vi "Grab Tool.vi"(8 "error in":errorcluster, 9 "Tool Type":enum16{"Stamp", "Weight"}(ring), 10 "Slot Number":i32, 11 "GrabberTool in":refnum<class "GrabberTool Class.lvclass">) -> (0 "error out":errorcluster, 3 "GrabberTool out":refnum<class "GrabberTool Class.lvclass">)   [LabVIEW 2011, in "GrabberTool Class.lvclass"]
uses:
  GrabberTool Class.lvclass
  Config Manager Class/Type Definitions/Part Type.ctl
  Config Manager Class/Type Definitions/Offset.ctl
  Config Manager Class/Type Definitions/Named Position.ctl
  WorkTable Class/WorkTable Class.lvclass
  Vec3d Class/Vec3d Class.lvclass
  Config Manager Class/Read Geometry Definition 3D.vi
  Config Manager Class/Config Manager Class.lvclass
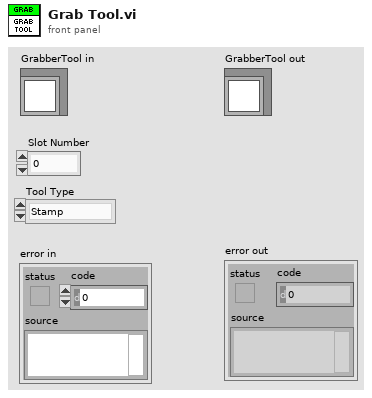
[diagram p1: front panel]
types:
  T1 = typedef "Part Type.ctl" = enum16{"BBM", "HDI", "BARE HDI", "GLUERESERVOIR", "STAMP_1", "STAMP_2", "STAMP_3", "STAMP_4", "STAMP_5", "WEIGHT_1", "WEIGHT_2", "WEIGHT_3", "WEIGHT_4", "WEIGHT_5", "WEIGHT_6", "WEIGHT_7", "WEIGHT_8", "PICKER_TOOL", "GRABER_TOOL"}
  T2 = typedef "Offset.ctl" = enum16{"needle_offset", "tool_holder_offset"}
  T3 = typedef "Named Position.ctl" = enum16{"home", "module_chuck_0", "module_chuck_1", "module_chuck_2", "module_chuck_3", "module_chuck_4", "glue_reservoir_chuck", "stamp_tool_chuck", "weight_tool_chuck", "needle_calibration", "tool_rack_pos_0_in", "tool_rack_pos_0_out", "tool_rack_pos_1_in", "tool_rack_pos_1_out", "tool_rack_pos_2_in", "tool_rack_pos_2_out", "front_load_position", "grabber_start_pos", "between_chuck_0_and_1", "between_chuck_2_and_3"}
  T4 = typedef "Worktable_Weights.ctl" = cluster{"Weight Slots":cluster{"Weight State":enum16{"Empty", "Populated"}, "Weight Type":T5, "Location/Orientation":T6}[], "Vacuum Channel":i32}
  T5 = typedef "Weight Type.ctl" = enum16{"Weight 1", "Weight 2", "Weight 3", "Weight 4", "Weight 5", "Weight 6", "Weight 7", "Weight 8"}
  T6 = typedef "Position_Orientation.ctl" = cluster{"Center":refnum<class "Vec3d Class.lvclass">, "Orientation":refnum<class "Orient3d Class.lvclass">}
  T7 = cluster{"Weight State":enum16{"Empty", "Populated"}, "Weight Type":T5, "Location/Orientation":T6}[]
  T8 = cluster{"Weight State":enum16{"Empty", "Populated"}, "Weight Type":T5, "Location/Orientation":T6}
  T9 = typedef "Worktable_Stamps.ctl" = cluster{"Stamp Slots":T10[], "Vacuum Channel":i32}
  T10 = typedef "Worktable_Stamp.ctl" = cluster{"Stamp State":enum16{"Empty", "Populated", "Used"}, "Location/Orientation":T6, "Stamp Type":T11}
  T11 = typedef "Stamp Type.ctl" = enum16{"Stamp 1", "Stamp 2", "Stamp 3", "Stamp 4", "Stamp 5"}
  T12 = typedef "Gluing Parameters.ctl" = cluster{"Safe Grabber Pickup":dbl, "Safe Grabber Lift":dbl, "Glue Resevoir Wait Time":dbl, "Glue BM Wait Time ":dbl, "Placed Weight X-Move":dbl}
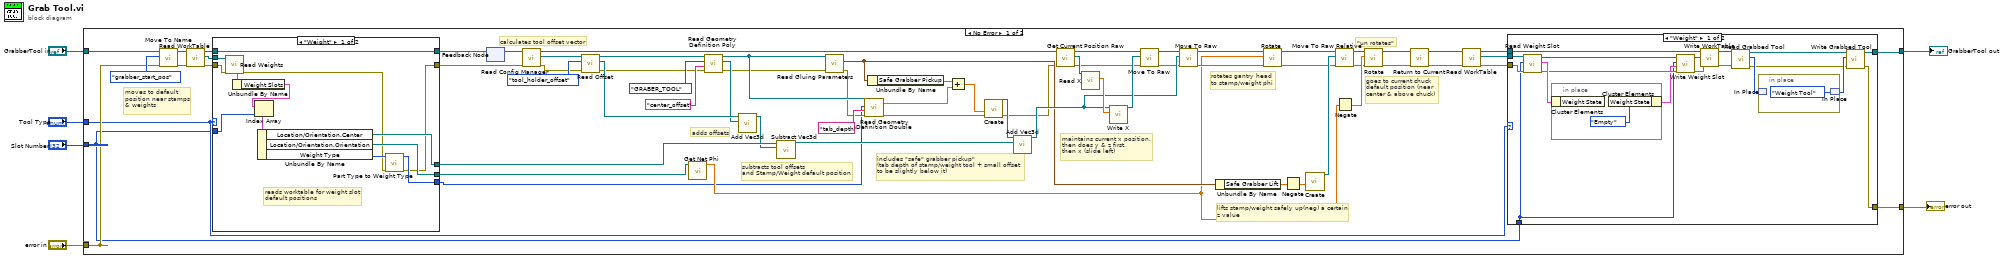
[diagram p0: block diagram]
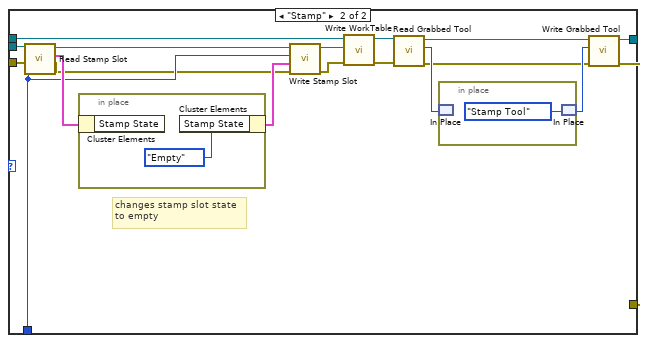
[diagram p2: hidden frame]
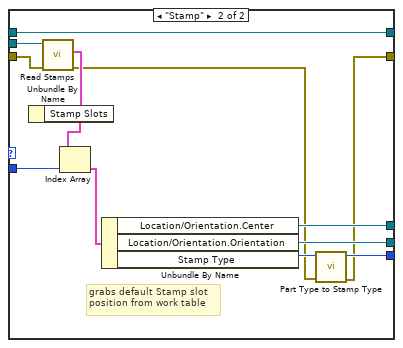
[diagram p3: hidden frame]
diagram:
  n1 = case shown="No Error" "error in" {
    selector: "error in" -> [w22 w139]
    tunnel: [w14 w139] -> w5
    tunnel: [w15 w140] -> w6
    tunnel: "GrabberTool in" -> [w71 w140]
    tunnel: "Slot Number" -> [w7 _]
    tunnel: [w22 w139] -> _
    tunnel: "Tool Type" -> [w8 _]
    frame No Error {
      # "includes \"safe\" grabber pickup\"\n(tab depth of stamp/weight tool + small offset \nto be slightly below it)"
      # "goes to current chuck\ndefault position (near\ncenter & above chuck)"
      # "\"un rotates\""
      # "lifts stamp/weight safely up(neg) a certain\nz value"
      # "rotates gantry head\nto stamp/weight phi"
      # "maintains current x position, \nthen does y & z first,\nthen x (slide left)"
      # "subtracts tool offsets\nand Stamp/Weight default position"
      # "adds offsets"
      # "calculates tool offset vector"
      # "moves to default\nposition near stamps\n& weights"
      n2 = call-dynamic "Move To Name.vi"("error in"=w22, "Destination"=Named_Position."grabber_start_pos", "Gantry in"=w71) -> ("error out"=w69:errorcluster, "Gantry out"=w68:refnum<class "GrabberTool Class.lvclass">)  [unwired: 7 in]
      n3 = call-dynamic "Read WorkTable.vi"("error in"=w69, "Gantry Class in"=w68) -> ("error out"=w30:errorcluster, "WorkTable Class.lvclass"=w67:refnum<class "WorkTable Class.lvclass">, "Gantry Class out"=w13:refnum<class "GrabberTool Class.lvclass">)  [unwired: 7 in]
      n4 = case shown="\"Weight\"" w8 {
        tunnel: [w117 w135] -> w70
        tunnel: w67 -> [w124 w134]
        tunnel: [w116 w133] -> w60
        tunnel: [w114 w127] -> w9
        tunnel: w30 -> [w123 w132]
        tunnel: [w118 w130] -> w21
        tunnel: w13 -> [w113 w129]
        tunnel: [w113 w129] -> w12
        tunnel: w7 -> [w120 w126]
        frame "Weight" {
          # "reads worktable for weight slot\ndefault positions"
          n5 = call-dynamic "Read Weights.vi"("error in (no error)"=w123, "WorkTable Class in"=w124) -> ("error out"=w115:errorcluster, "Weights"=w122:T4)  [unwired: 7 in, 1 out]
          n6 = Unbundle By Name(w122) -> ("Weight Slots"=w121:T7)
          n7 = Index Array(array=w121, index=w120) -> (element=w119:T8)
          n8 = Unbundle By Name(w119) -> ("Location/Orientation.Center"=w116:refnum<class "Vec3d Class.lvclass">, "Location/Orientation.Orientation"=w117:refnum<class "Orient3d Class.lvclass">, "Weight Type"=w125:T5)
          n9 = call "Part Type to Weight Type.vi"("error in"=w115, "Weight Type"=w125) -> ("error out"=w114:errorcluster, "Part Type"=w118:T1)  [unwired: 8 in]
        }
        frame "Stamp" {
          # "grabs default Stamp slot\nposition from work table"
          n10 = call-dynamic "Read Stamps.vi"("error in (no error)"=w132, "WorkTable Class in"=w134) -> ("error out"=w128:errorcluster, "Stamps"=w138:T9)  [unwired: 7 in, 1 out]
          n11 = Unbundle By Name(w138) -> ("Stamp Slots"=w137:T10[])
          n12 = Index Array(array=w137, index=w126) -> (element=w136:T10)
          n13 = Unbundle By Name(w136) -> ("Location/Orientation.Center"=w133:refnum<class "Vec3d Class.lvclass">, "Location/Orientation.Orientation"=w135:refnum<class "Orient3d Class.lvclass">, "Stamp Type"=w131:T11)
          n14 = call "Part Type to Stamp Type.vi"("error in"=w128, "Stamp Type"=w131) -> ("error out"=w127:errorcluster, "Part Type"=w130:T1)  [unwired: 8 in]
        }
      }
      n15 = feedback-in #1(w12) -> ()
      n16 = feedback #1() -> (w11:refnum<class "GrabberTool Class.lvclass">)  [unwired: 1 in]
      n17 = call-dynamic "Read Config Manager.vi"("error in"=w9, "Gantry in"=w11) -> ("error out"=w31:errorcluster, "Config Manager"=w65:refnum<class "Config Manager Class.lvclass">, "Gantry out"=w51:refnum<class "GrabberTool Class.lvclass">)  [unwired: 7 in]
      n18 = call "Read Offset.vi"("error in"=w31, "Offset"=Offset."tool_holder_offset", "Config Manager in"=w65) -> ("error out"=w10:errorcluster, "Vec3d out"=w62:refnum<class "Vec3d Class.lvclass">, "Config Manager out"=w24:refnum<class "Config Manager Class.lvclass">)  [unwired: 6 in]
      n19 = call "Get Net Phi.vi"("Orient3d"=w70) -> ("phi(deg)"=w23:dbl)  [unwired: 8 in, 2 out]
      n20 = call-poly "Read Geometry Definition Poly.vi"("error in"=w10, "Feature"="center_offset", "Part Type"=Part_Type."GRABER_TOOL", "Config Manager in"=w24) -> ("error out"=w32:errorcluster, "Feature Coordinates"=w61:refnum<class "Vec3d Class.lvclass">, "Config Manager out"=w58:refnum<class "Config Manager Class.lvclass">)  [unwired: 5 in]
      n21 = call-dynamic "Add Vec3d.vi"(10:"Vec3d Class in"=w61, 11:"Vec3d Class in"=w62) -> ("Vec3d Class out"=w59:refnum<class "Vec3d Class.lvclass">)  [unwired: 8 in, 1 out]
      n22 = call "Subtract Vec3d.vi"("Vec3d in 2"=w59, "Vec3d in 1"=w60) -> ("Vec3d Class out"=w52:refnum<class "Vec3d Class.lvclass">)  [unwired: 8 in, 1 out]
      n23 = call "Read Gluing Parameters.vi"("error in (no error)"=w32, "Config Manager Class in"=w58) -> ("error out"=w33:errorcluster, "Gluing Parameters"=w43:T12)  [unwired: 7 in, 1 out]
      n24 = call "Read Geometry Definition Double.vi"("error in"=w33, "Feature"="tab_depth", "Part Type"=w21, "Config Manager in"=w58) -> ("error out"=w34:errorcluster, "Geometry Definition"=w55:dbl)  [unwired: 5 in, 1 out]
      n25 = Unbundle By Name(w43) -> ("Safe Grabber Pickup"=w56:dbl)
      n26 = Add(x=w56, y=w55) -> (x+y=w54:dbl)
      n27 = call "Create.vi"("Z"=w54) -> ("Vec3d Class out"=w53:refnum<class "Vec3d Class.lvclass">)  [unwired: 9 in, 1 out]
      n28 = call-dynamic "Add Vec3d.vi"(10:"Vec3d Class in"=w52, 11:"Vec3d Class in"=w53) -> ("Vec3d Class out"=w46:refnum<class "Vec3d Class.lvclass">)  [unwired: 8 in, 1 out]
      n29 = call-dynamic "Get Current Position Raw.vi"("error in"=w34, "Gantry in"=w51) -> ("error out"=w35:errorcluster, "Vec3d Class out"=w50:refnum<class "Vec3d Class.lvclass">, "Gantry out"=w48:refnum<class "GrabberTool Class.lvclass">)  [unwired: 7 in]
      n30 = call-dynamic "Read X.vi"("Vec3d Class in"=w50) -> ("X"=w49:dbl)  [unwired: 8 in, 2 out]
      n31 = call-dynamic "Write X.vi"("X"=w49, "Vec3d Class in"=w46) -> ("Vec3d Class out"=w47:refnum<class "Vec3d Class.lvclass">)  [unwired: 8 in, 1 out]
      n32 = call-dynamic "Move To Raw.vi"("error in"=w35, "Destination"=w47, "Gantry in"=w48) -> ("error out"=w36:errorcluster, "Gantry out"=w45:refnum<class "GrabberTool Class.lvclass">)  [unwired: 7 in]
      n33 = call-dynamic "Move To Raw.vi"("error in"=w36, "Destination"=w46, "Gantry in"=w45) -> ("error out"=w37:errorcluster, "Gantry out"=w44:refnum<class "GrabberTool Class.lvclass">)  [unwired: 7 in]
      n34 = Unbundle By Name(w43) -> ("Safe Grabber Lift"=w42:dbl)
      n35 = call-dynamic "Rotate.vi"("error in"=w37, "distance(deg)"=w23, "Gantry in"=w44) -> ("error out"=w38:errorcluster, "Gantry out"=w39:refnum<class "GrabberTool Class.lvclass">)  [unwired: 7 in]
      n36 = Negate(x=w42) -> (-x=w41:dbl)
      n37 = call "Create.vi"("Z"=w41) -> ("Vec3d Class out"=w40:refnum<class "Vec3d Class.lvclass">)  [unwired: 9 in, 1 out]
      n38 = call-dynamic "Move To Raw Relative.vi"("error in"=w38, "Delta"=w40, "Gantry in"=w39) -> ("error out"=w27:errorcluster, "Gantry out"=w28:refnum<class "GrabberTool Class.lvclass">)  [unwired: 7 in]
      n39 = Negate(x=w23) -> (-x=w29:dbl)
      n40 = call-dynamic "Rotate.vi"("error in"=w27, "distance(deg)"=w29, "Gantry in"=w28) -> ("error out"=w25:errorcluster, "Gantry out"=w26:refnum<class "GrabberTool Class.lvclass">)  [unwired: 7 in]
      n41 = call-dynamic "Return to Current.vi"("error in"=w25, "Gantry in"=w26) -> ("error out"=w19:errorcluster, "Gantry out"=w20:refnum<class "GrabberTool Class.lvclass">)  [unwired: 8 in]
      n42 = call-dynamic "Read WorkTable.vi"("error in"=w19, "Gantry Class in"=w20) -> ("error out"=w17:errorcluster, "WorkTable Class.lvclass"=w18:refnum<class "WorkTable Class.lvclass">, "Gantry Class out"=w16:refnum<class "GrabberTool Class.lvclass">)  [unwired: 7 in]
      n43 = case shown="\"Weight\"" w8 {
        tunnel: w18 -> [w83 w110]
        tunnel: w7 -> [w81 w108]
        tunnel: w17 -> [w82 w105]
        tunnel: w16 -> [w84 w103]
        tunnel: [w74 w96] -> w15
        tunnel: [w73 w93] -> w14
        frame "Weight" {
          n44 = call "Read Weight Slot.vi"("error in (no error)"=w82, "weight slot"=w81, "WorkTable Class in"=w83) -> ("error out"=w88:errorcluster, "Weight Slot"=w90:T8, "WorkTable Class out"=w89:refnum<class "WorkTable Class.lvclass">)  [unwired: 6 in]
          n45 = in-place {
            n46 = in-place-cluster #2(w90) -> ()  [unwired: 1 out]
            n47 = in-place-cluster #2("Weight State"=enum16{"Empty", "Populated", "Used"}."Empty" ("Stamp State")) -> (w87:T8)
          }
          n48 = call "Write Weight Slot.vi"("error in (no error)"=w88, "Weight Slot"=w87, "weight slot"=w81, "WorkTable Class in"=w89) -> ("error out"=w85:errorcluster, "WorkTable Class out"=w86:refnum<class "WorkTable Class.lvclass">)  [unwired: 6 in]
          n49 = call-dynamic "Write WorkTable.vi"("error in (no error)"=w85, "WorkTable Class.lvclass"=w86, "Gantry Class in"=w84) -> ("error out"=w75:errorcluster, "Gantry Class out"=w76:refnum<class "GrabberTool Class.lvclass">)  [unwired: 7 in]
          n50 = call "Read Grabbed Tool.vi"("error in (no error)"=w75, "GrabberTool Class in"=w76) -> ("error out"=w77:errorcluster, "Grabbed Tool"=w80:enum16{"Weight Tool", "Stamp Tool", "Nothing"}, "GrabberTool Class out"=w78:refnum<class "GrabberTool Class.lvclass">)  [unwired: 7 in]
          n51 = in-place {
            n52 = in-place-match #3(w80) -> ()  [unwired: 1 out]
            n53 = in-place-match #3(enum16{"Weight Tool", "Stamp Tool", "Nothing"}."Weight Tool" ("Grabbed Tool")) -> (w79:enum16{"Weight Tool", "Stamp Tool", "Nothing"})
          }
          n54 = call "Write Grabbed Tool.vi"("error in (no error)"=w77, "Grabbed Tool"=w79, "GrabberTool Class in"=w78) -> ("error out"=w73:errorcluster, "GrabberTool Class out"=w74:refnum<class "GrabberTool Class.lvclass">)  [unwired: 7 in]
        }
        frame "Stamp" {
          # "changes stamp slot state\nto empty"
          n55 = call "Read Stamp Slot.vi"("error in (no error)"=w105, "Stamp Slot"=w108, "WorkTable Class in"=w110) -> ("error out"=w104:errorcluster, "Stamp Slot"=w109:T10, "WorkTable Class out"=w106:refnum<class "WorkTable Class.lvclass">)  [unwired: 6 in]
          n56 = in-place {
            n57 = in-place-cluster #4(w109) -> ()  [unwired: 1 out]
            n58 = in-place-cluster #4("Stamp State"=enum16{"Empty", "Populated", "Used"}."Empty") -> (w107:T10)
          }
          n59 = call "Write Stamp Slot.vi"("error in (no error)"=w104, 9:"Stamp Slot"=w107, 10:"Stamp Slot"=w108, "WorkTable Class in"=w106) -> ("error out"=w101:errorcluster, "WorkTable Class out"=w102:refnum<class "WorkTable Class.lvclass">)  [unwired: 6 in]
          n60 = call-dynamic "Write WorkTable.vi"("error in (no error)"=w101, "WorkTable Class.lvclass"=w102, "Gantry Class in"=w103) -> ("error out"=w95:errorcluster, "Gantry Class out"=w100:refnum<class "GrabberTool Class.lvclass">)  [unwired: 7 in]
          n61 = call "Read Grabbed Tool.vi"("error in (no error)"=w95, "GrabberTool Class in"=w100) -> ("error out"=w94:errorcluster, "Grabbed Tool"=w99:enum16{"Weight Tool", "Stamp Tool", "Nothing"}, "GrabberTool Class out"=w97:refnum<class "GrabberTool Class.lvclass">)  [unwired: 7 in]
          n62 = in-place {
            n63 = in-place-match #5(w99) -> ()  [unwired: 1 out]
            n64 = in-place-match #5(enum16{"Weight Tool", "Stamp Tool", "Nothing"}."Stamp Tool" ("Grabbed Tool")) -> (w98:enum16{"Weight Tool", "Stamp Tool", "Nothing"})
          }
          n65 = call "Write Grabbed Tool.vi"("error in (no error)"=w94, "Grabbed Tool"=w98, "GrabberTool Class in"=w97) -> ("error out"=w93:errorcluster, "GrabberTool Class out"=w96:refnum<class "GrabberTool Class.lvclass">)  [unwired: 7 in]
        }
      }
    }
    frame Error {
    }
  }
  "GrabberTool out" <- w6
  "error out" <- w5
